vi "Write Slices and Colors.vi"(8 "error in (no error)":errorcluster, 10 "Slices and Colors[]":T1[](array[typedef]), 11 "PieChart in":refnum<class "PieChart.lvclass">) -> (0 "error out":errorcluster, 3 "PieChart out":refnum<class "PieChart.lvclass">)   [LabVIEW 2018, in "PieChart.lvclass"]
uses:
  PieChart.lvclass
  Pie Slice with Color.ctl
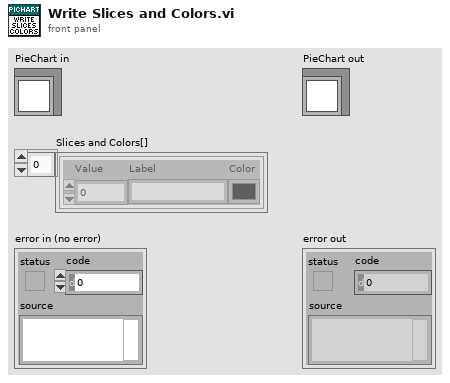
[diagram p1: front panel]
types:
  T1 = typedef "PieChart.lvclass/Pie Slice with Color.ctl" = cluster{"Value":dbl, "Label":string, "Color":u32}
  T2 = typedef "PieChart.lvclass/State Data.ctl" = cluster{"Title":string, "Values[]":dbl[], "Labels[]":string[], "Colors[]":u32[], "Include Legend?":bool, "Include Title?":bool, "Title Font":T3, "Legend Font":T3, "Selection":i32, "Slice Positions":T4}
  T3 = typedef "LVFontTypeDef.ctl" = cluster{"Font Name":string, "Size":u16, "Bold":bool, "Italic":bool, "Underline":bool, "Strikeout":bool, "Color":u32}
  T4 = typedef "PieChart.lvclass/Pie info for Click.ctl" = cluster{"Slice Positions":cluster{"Start":i16, "End":i16}[], "Center Position":T5, "Radius":i16}
  T5 = typedef "LVBoundsTypeDef.ctl" = cluster{"Width":u32, "Height":u32}
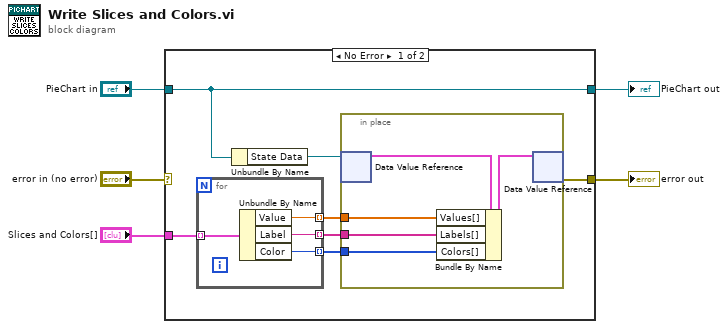
[diagram p0: block diagram]
diagram:
  n1 = case shown="No Error" "error in (no error)" {
    selector: "error in (no error)" -> [_ w23]
    tunnel: [w10 w23] -> w4
    tunnel: [w11 w22] -> w2
    tunnel: "PieChart in" -> [w11 w22]
    tunnel: "Slices and Colors[]" -> [w9 _]
    frame No Error {
      n2 = for {
        tunnel: w9 -> [w16] mode=indexing
        tunnel: [w15] -> w8 mode=indexing
        tunnel: [w14] -> w7 mode=indexing
        tunnel: [w13] -> w6 mode=indexing
        n3 = Unbundle By Name(w16) -> ("Value"=w15:dbl, "Label"=w14:string, "Color"=w13:u32)
      }
      n4 = Unbundle By Name(w11) -> ("State Data"=w12:refnum<data-value>)
      n5 = in-place {
        in-place-border: w8 -> [w19]
        in-place-border: w7 -> [w18]
        in-place-border: w6 -> [w17]
        n6 = in-place-dvr #1(w12) -> (w21:T2)  [unwired: 1 out]
        n7 = Bundle By Name(cluster=w21, "Values[]"=w19, "Labels[]"=w18, "Colors[]"=w17) -> (w20:T2)
        n8 = in-place-dvr #1(w20) -> (w10:errorcluster)  [unwired: 1 out]
      }
    }
    frame Error {
    }
  }
  "error out" <- w4
  "PieChart out" <- w2
